vi "Open.vi"(7 "Config data in":variant, 8 "error in (no error)":errorcluster, 9 "Timeout (ms)":u32=3000, 10 "VISA session":refnum<visa-resource-name>="TCPIP::146.201.232.88::7180::SOCKET", 11 "PS Driver AMI4xx.lvlib:PS Driver AMI4xx.lvclass in":refnum<class "PS Driver AMI4xx.lvclass">) -> (0 "error out":errorcluster, 1 "Config data out":variant, 2 "dup VISA Session":refnum<visa-resource-name>, 3 "PS Driver AMI4xx.lvlib:PS Driver AMI4xx.lvclass out":refnum<class "PS Driver AMI4xx.lvclass">)   [LabVIEW 2025, in "PS Driver.lvlib" / "PS Driver AMI4xx.lvclass"]
doc: "Author: Scott Hannahs <sth@magnet.fsu.edu>\n\nThis software is licensed for use under the “MIT License\"\nCopyright (c) 2025 Scott Hannahs, sth@sth@magnet.sthnet.net\n\nPermission is hereby granted, free of charge, to any person obtaining a copy of this software and associated documentation files (the \"Software\"), to deal in the Software without restriction, including without limitation the rights to use, copy, modify, merge, publish, distribute, sublicense, and/or sell copies of the Software, and to permit persons to whom the Software is furnished to do so, subject to the following conditions: The above copyright notice and this permission notice shall be included in all copies or substantial portions of the Software.\n\nTHE SOFTWARE IS PROVIDED \"AS IS\", WITHOUT WARRANTY OF ANY KIND, EXPRESS OR IMPLIED, INCLUDING BUT NOT LIMITED TO THE WARRANTIES OF MERCHANTABILITY, FITNESS FOR A PARTICULAR PURPOSE AND NONINFRINGEMENT. IN NO EVENT SHALL THE AUTHORS OR COPYRIGHT HOLDERS BE LIABLE FOR ANY CLAIM, DAMAGES OR OTHER LIABILITY, WHETHER IN AN ACTION OF CONTRACT, TORT OR OTHERWISE, ARISING FROM, OUT OF OR IN CONNECTION WITH THE SOFTWARE OR THE USE OR OTHER DEALINGS IN THE SOFTWARE."
uses:
  PS Driver AMI4xx.lvclass
  PS Driver.lvclass/PS Driver.ctl
  PS Driver with Persistence.lvclass
  PS Driver.lvclass
panel:
  out "IDN string":string
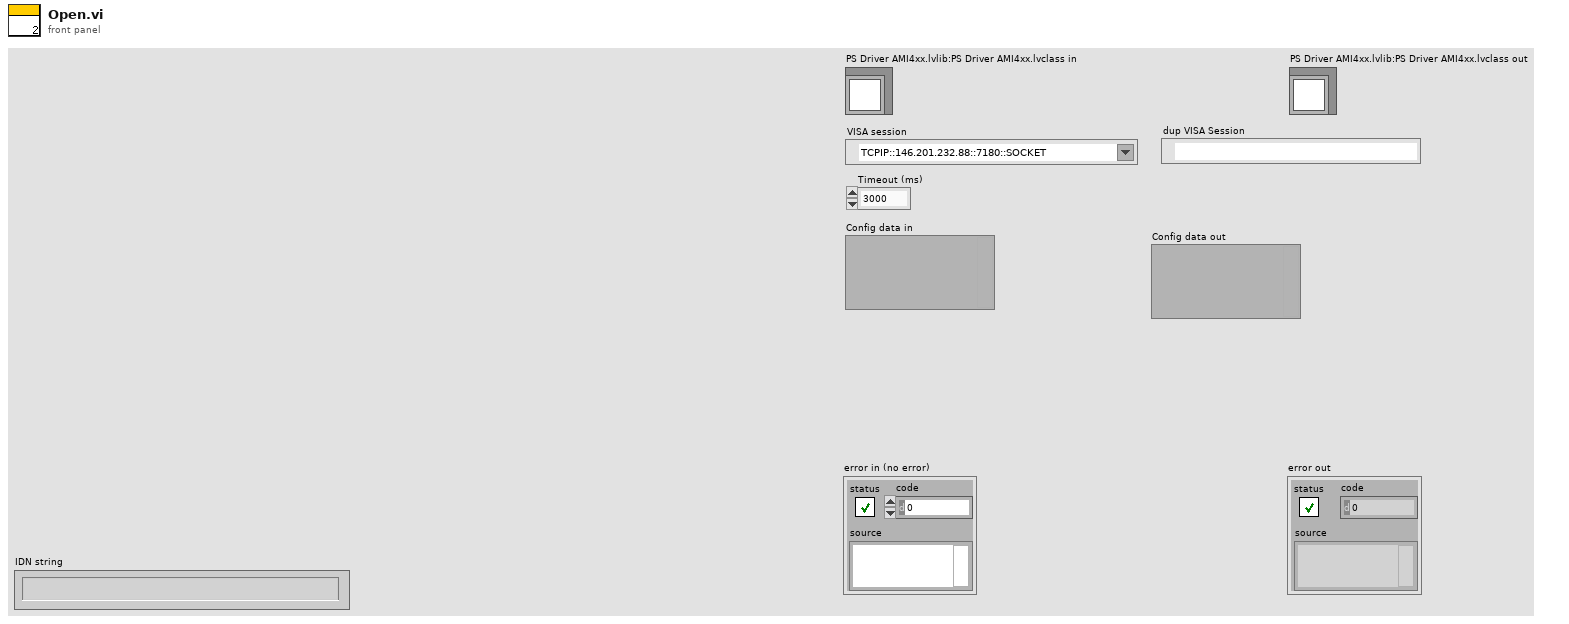
[diagram p1: front panel]
types:
  T1 = cluster{"INI key name":string, "Configuration command":string}[]
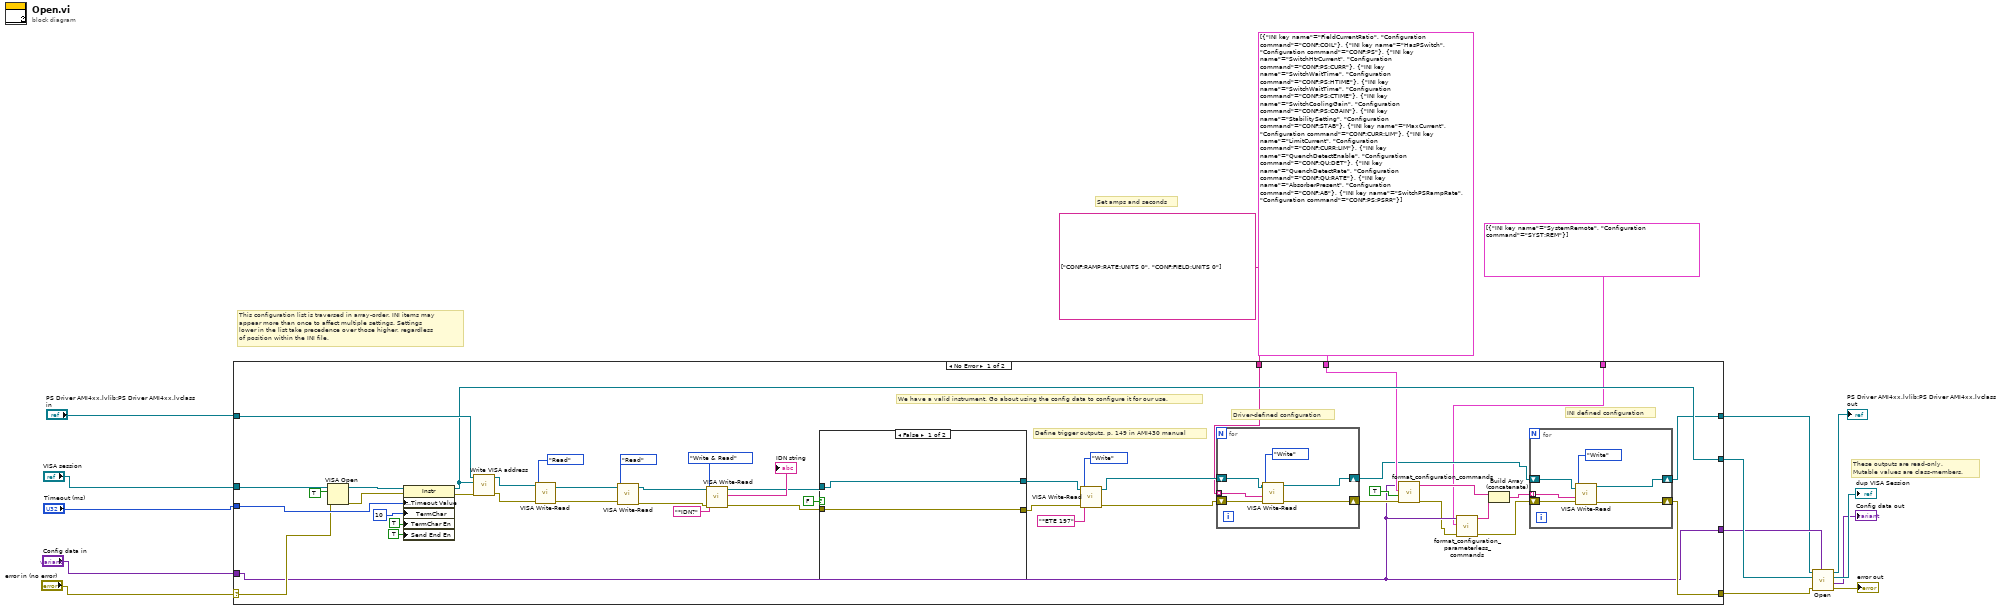
[diagram p0: block diagram]
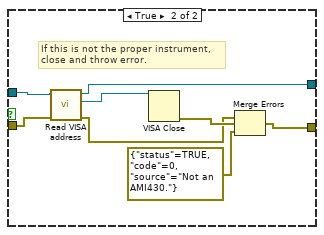
[diagram p2: hidden frame]
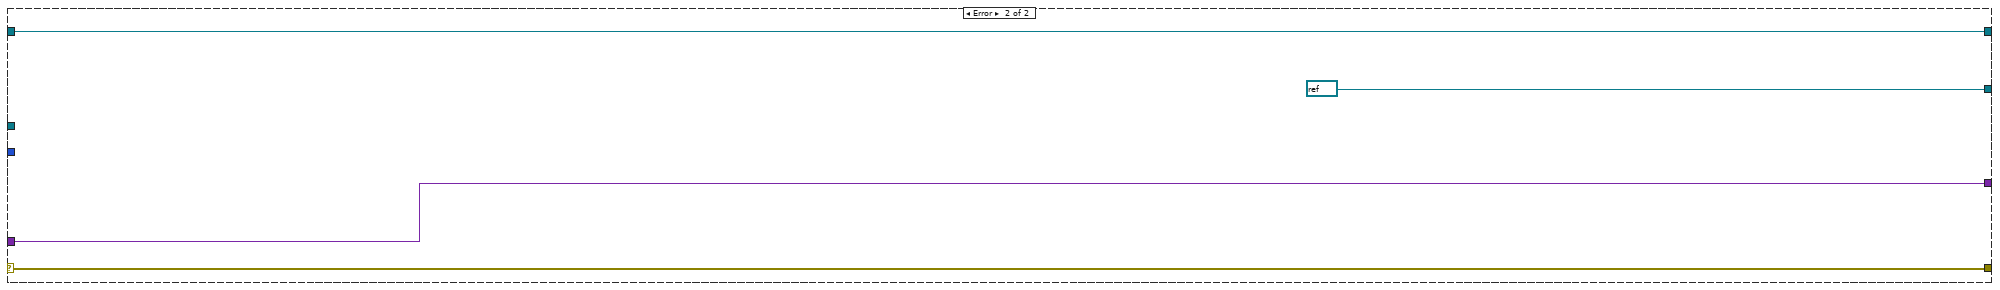
[diagram p3: hidden frame]
diagram:
  # "Set amps and seconds"
  # "These outputs are read-only.\nMutable values are class-members."
  # "This configuration list is traversed in array-order. INI items may\nappear more than once to affect multiple settings. Settings\nlower in the list take precedence over those higher, regardless\nof position within the INI file."
  n1 = case shown="No Error" "error in (no error)" {
    selector: "error in (no error)" -> [w54 w88]
    tunnel: [w28 w88] -> w15
    tunnel: [w29 w87] -> w12
    tunnel: "PS Driver AMI4xx.lvlib:PS Driver AMI4xx.lvclass in" -> [w40 w87]
    tunnel: "VISA session" -> [w56 _]
    tunnel: "Timeout (ms)" -> [w55 _]
    tunnel: "Config data in" -> [w22 w85]
    tunnel: [w33 refnum<visa-resource-name> refnum ("dup VISA Session")] -> w16
    tunnel: [w22 w85] -> w13
    tunnel: T1 [{"INI key name"="FieldCurrentRatio", "Configuration command"="CONF:COIL"}, {"INI key name"="HasPSwitch", "Configuration command"="CONF:PS"}, {"INI key name"="SwitchHtrCurrent", "Configuration command"="CONF:PS:CURR"}, {"INI key name"="SwitchWaitTime", "Configuration command"="CONF:PS:HTIME"}, {"INI key name"="SwitchWaitTime", "Configuration command"="CONF:PS:CTIME"}, {"INI key name"="SwitchCoolingGain", "Configuration command"="CONF:PS:CGAIN"}, {"INI key name"="StabilitySetting", "Configuration command"="CONF:STAB"}, {"INI key name"="MaxCurrent", "Configuration command"="CONF:CURR:LIM"}, {"INI key name"="LimitCurrent", "Configuration command"="CONF:CURR:LIM"}, {"INI key name"="QuenchDetectEnable", "Configuration command"="CONF:QU:DET"}, {"INI key name"="QuenchDetectRate", "Configuration command"="CONF:QU:RATE"}, {"INI key name"="AbsorberPresent", "Configuration command"="CONF:AB"}, {"INI key name"="SwitchPSRampRate", "Configuration command"="CONF:PS:PSRR"}] -> [w32 _]
    tunnel: string[] ["CONF:RAMP:RATE:UNITS 0", "CONF:FIELD:UNITS 0"] -> [w23 _]
    tunnel: T1 [{"INI key name"="SystemRemote", "Configuration command"="SYST:REM"}] -> [w19 _]
    frame No Error {
      # "Driver-defined configuration"
      # "INI defined configuration"
      # "Define trigger outputs. p. 149 in AMI430 manual"
      # "We have a valid instrument. Go about using the config data to configure it for our use."
      n2 = VISA Open(duplicate session (F)=TRUE, error in (no error)=w54, VISA resource name=w56) -> (VISA resource name=w62:refnum<visa-resource-name>, error out=w60:errorcluster)  [unwired: 2 in]
      n3 = property class="Instr"(reference=w62, error in=w60, "General Settings:Timeout Value"=w55, "TermChar"=u8 10 ("Message Based Settings:Termination Character"), "TermChar En"=TRUE ("Message Based Settings:Termination Character Enable"), "Send End En"=TRUE ("Message Based Settings:Send End Enable")) -> (reference out=w33:refnum<visa-resource-name>, error out=w41:errorcluster)
      n4 = call "Write VISA address.vi"("error in (no error)"=w41, "VISA address"=w33, "PS Driver in"=w40) -> ("error out"=w38:errorcluster, "PS Driver out"=w39:refnum<class "PS Driver AMI4xx.lvclass">)  [unwired: 7 in]
      n5 = call "VISA Write-Read.vi"("error in (no error)"=w38, "Action"=enum16{"Write", "Read", "Write & Read"}."Read", "PS Driver.lvlib:PS Driver AMI4xx.lvclass"=w39) -> ("error out"=w42:errorcluster, "PS Driver.lvlib:PS Driver AMI4xx.lvclass out"=w43:refnum<class "PS Driver AMI4xx.lvclass">)  [unwired: 5 in, 2 out]
      n6 = call "VISA Write-Read.vi"("error in (no error)"=w42, "Action"=enum16{"Write", "Read", "Write & Read"}."Read", "PS Driver.lvlib:PS Driver AMI4xx.lvclass"=w43) -> ("error out"=w44:errorcluster, "PS Driver.lvlib:PS Driver AMI4xx.lvclass out"=w45:refnum<class "PS Driver AMI4xx.lvclass">)  [unwired: 5 in, 2 out]
      n7 = call "VISA Write-Read.vi"("error in (no error)"=w44, "Command String"="*IDN?", "Action"=enum16{"Write", "Read", "Write & Read"}."Write & Read", "PS Driver.lvlib:PS Driver AMI4xx.lvclass"=w45) -> ("error out"=w48:errorcluster, "Response string"=→"IDN string":string, "PS Driver.lvlib:PS Driver AMI4xx.lvclass out"=w46:refnum<class "PS Driver AMI4xx.lvclass">)  [unwired: 4 in, 1 out]
      n8 = case shown="False" FALSE {
        tunnel: w48 -> [w76 w79]
        tunnel: [w76 w82] -> w35
        tunnel: [w75 w80] -> w34
        tunnel: w46 -> [w75 w77]
        frame False {
        }
        frame True {
          # "If this is not the proper instrument,\nclose and throw error."
          n9 = call "Read VISA address.vi"("error in (no error)"=w79, "PS Driver in"=w77) -> ("error out"=w78:errorcluster, "VISA address"=w81:refnum<visa-resource-name>, "PS Driver out"=w80:refnum<class "PS Driver AMI4xx.lvclass">)  [unwired: 7 in]
          n10 = VISA Close(VISA resource name=w81) -> (error out=w84:errorcluster)  [unwired: 1 in]
          n11 = Merge Errors(w78, w84, errorcluster {"status"=TRUE, "code"=0, "source"="Not an AMI430."} ("error IO")) -> (w82:errorcluster)
        }
      }
      n12 = call "VISA Write-Read.vi"("error in (no error)"=w35, "Command String"="*ETE 197", "Action"=enum16{"Write", "Read", "Write & Read"}."Write", "PS Driver.lvlib:PS Driver AMI4xx.lvclass"=w34) -> ("error out"=w26:errorcluster, "PS Driver.lvlib:PS Driver AMI4xx.lvclass out"=w27:refnum<class "PS Driver AMI4xx.lvclass">)  [unwired: 4 in, 2 out]
      n13 = for {
        shift-right: [w63] -> w25
        shift-left: w26 -> [w66]
        shift-right: [w64] -> w24
        shift-left: w27 -> [w67]
        tunnel: w23 -> [w65] mode=indexing
        n14 = call "VISA Write-Read.vi"("error in (no error)"=w66, "Command String"=w65, "Action"=enum16{"Write", "Read", "Write & Read"}."Write", "PS Driver.lvlib:PS Driver AMI4xx.lvclass"=w67) -> ("error out"=w63:errorcluster, "PS Driver.lvlib:PS Driver AMI4xx.lvclass out"=w64:refnum<class "PS Driver AMI4xx.lvclass">)  [unwired: 4 in, 2 out]
      }
      n15 = call "format_configuration_commands.vi"("error in (no error)"=w25, "True/false to 0/1?"=TRUE, "Configuration editables"=w32, "Config data in"=w22) -> ("error out"=w21:errorcluster, "Configuration commands"=w30:string[])  [unwired: 6 in]
      n16 = call "format_configuration_parameterless_commands.vi"("error in (no error)"=w21, "Configuration editables"=w19, "Config data in"=w22) -> ("error out"=w20:errorcluster, "Configuration commands"=w17:string[])  [unwired: 7 in]
      n17 = Build Array (concatenate)(w30, w17) -> (w18:string[])
      n18 = for {
        shift-right: [w69] -> w28
        shift-left: w20 -> [w72]
        shift-right: [w70] -> w29
        shift-left: w24 -> [w73]
        tunnel: w18 -> [w71] mode=indexing
        n19 = call "VISA Write-Read.vi"("error in (no error)"=w72, "Command String"=w71, "Action"=enum16{"Write", "Read", "Write & Read"}."Write", "PS Driver.lvlib:PS Driver AMI4xx.lvclass"=w73) -> ("error out"=w69:errorcluster, "PS Driver.lvlib:PS Driver AMI4xx.lvclass out"=w70:refnum<class "PS Driver AMI4xx.lvclass">)  [unwired: 4 in, 2 out]
      }
    }
    frame Error {
    }
  }
  n20 = call-parent "Open.vi"("Config data in"=w13, "error in (no error)"=w15, "VISA session"=w16, "PS Driver.lvlib:PS Driver.lvclass in"=w12) -> ("error out"=→"error out":errorcluster, "Config data out"=→"Config data out":variant, "dup VISA Session"=→"dup VISA Session":refnum<visa-resource-name>, "PS Driver.lvlib:PS Driver.lvclass out"=→"PS Driver AMI4xx.lvlib:PS Driver AMI4xx.lvclass out":refnum<class "PS Driver AMI4xx.lvclass">)  [unwired: 4 in]
